vi "Tag Channel Example - Actually Right.vi"() -> ()   [LabVIEW 2023]
doc: "This VI demonstrates the fixes needed for the bugs that exist in the <b>Tag Channel Example - Almost Right.vi</b>."
uses:
  <extravilib>/ChannelInstances/Tag-u32/Instantiate.vi
  <extravilib>/ChannelInstances/Tag-u32/Endpoint.vi
  <extravilib>/ChannelInstances/Tag-u32/EndpointRead.vi
  <extravilib>/ChannelInstances/Tag-u32.lvlib
panel:
  out "C above threshold?":bool
  out "Thermometer C":dbl(slide) scale=0.0..10.0
  out "B above threshold?":bool
  out "Thermometer B":dbl(slide) scale=0.0..10.0
  out "A above threshold?":bool
  out "Thermometer A":dbl(slide) scale=0.0..10.0
  in  "Threshold Setting":u32(slide)=5 scale=0.0..10.0
  in  "Stop":bool
  # "Overview: Please review Tag Channel Example - Almost Right.vi before reviewing this VI.\n\nThis VI is identical to the other VI but with the two bugs fixed.\n\nInstructions:\n1. Run the VI. \n2. While running, change the Threshold Setting. Notice the thermometers immediately start using the new setting for their \"Too Hot\" indicators.\n3. Press the Stop button.\n4. Review the comments on the block diagram."
  # "When this VI is running, any time a thermometer is warmer than the Threshold Setting, that thermometer should say \"Too hot!\" in the Boolean at the bottom."
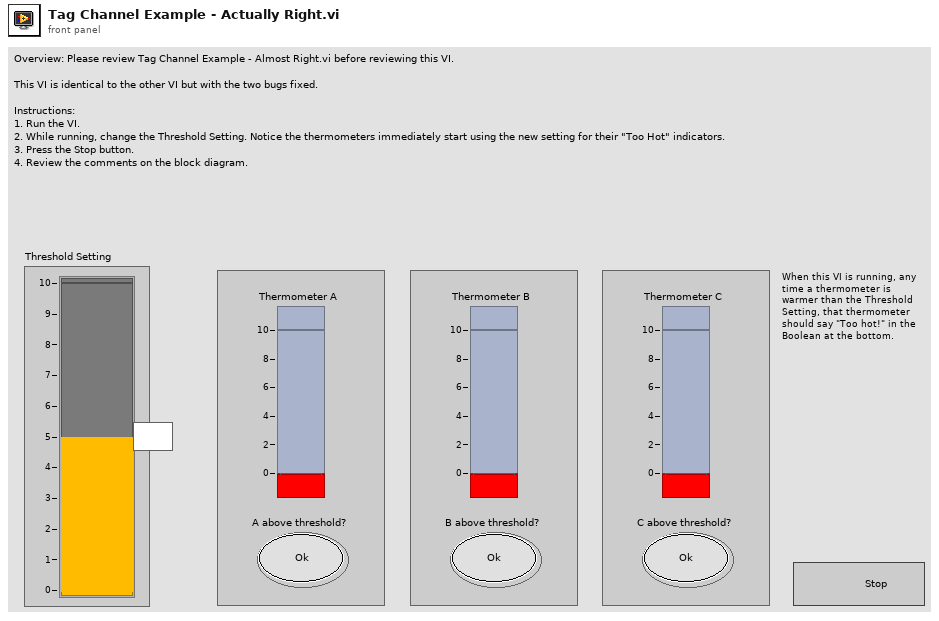
[diagram p1: front panel]
types:
  T1 = typedef "Tag-u32.lvlib/))Channel.ctl" = refnum<queue>
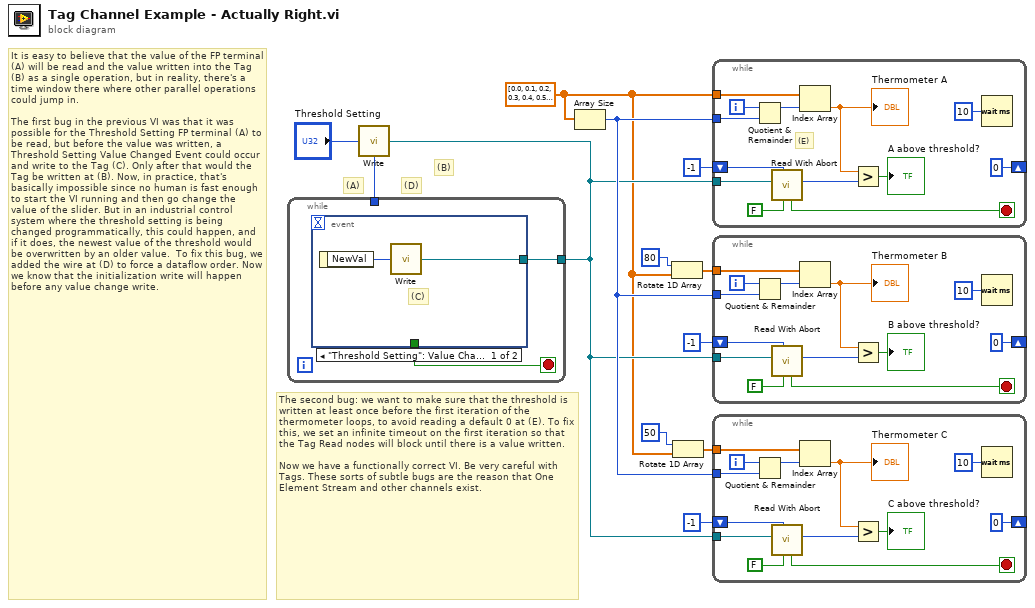
[diagram p0: block diagram]
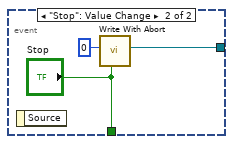
[diagram p2: hidden frame]
diagram:
  w7 = dbl[] [0.0, 0.1, 0.2, 0.3, 0.4, 0.5, 0.6, 0.7, 0.8, 0.9, 1.0, 1.1, 1.2, 1.3, 1.4, 1.5, 1.6, 1.7, 1.8, 1.9, 2.0, 2.1, 2.2, 2.3, 2.4, 2.5, 2.6, 2.7, 2.8, 2.9, 3.0, 3.1, 3.2, 3.3, 3.4, 3.5, 3.6, 3.7, 3.8, 3.9, 4.0, 4.1, 4.2, 4.3, 4.4, 4.5, 4.6, 4.7, 4.8, 4.9, 5.0, 5.1, 5.2, 5.3, 5.4, 5.5, 5.6, 5.7, 5.8, 5.9, 6.0, 6.1, 6.2, 6.3, 6.4, 6.5, 6.6, 6.7, 6.8, 6.9, 7.0, 7.1, 7.2, 7.3, 7.4, 7.5, 7.6, 7.7, 7.8, 7.9, 8.0, 8.1, 8.2, 8.3, 8.4, 8.5, 8.6, 8.7, 8.8, 8.9, 9.0, 9.1, 9.2, 9.3, 9.4, 9.5, 9.6, 9.7, 9.8, 9.9, 10.0, 10.0, 9.9, 9.8, 9.7, 9.6, 9.5, 9.4, 9.3, 9.2, 9.1, 9.0, 8.9, 8.8, 8.7, 8.6, 8.5, 8.4, 8.3, 8.2, 8.1, 8.0, 7.9, 7.8, 7.7, 7.6, 7.5, 7.4, 7.3, 7.2, 7.1, 7.0, 6.9, 6.8, 6.7, 6.6, 6.5, 6.4, 6.3, 6.2, 6.1, 6.0, 5.9, 5.8, 5.7, 5.6, 5.5, 5.4, 5.3, 5.2, 5.1, 5.0, 4.9, 4.8, 4.7, 4.6, 4.5, 4.4, 4.3, 4.2, 4.1, 4.0, 3.9, 3.8, 3.7, 3.6, 3.5, 3.4, 3.3, 3.2, 3.1, 3.0, 2.9, 2.8, 2.7, 2.6, 2.5, 2.4, 2.3, 2.2, 2.1, 2.0, 1.9, 1.8, 1.7, 1.6, 1.5, 1.4, 1.3, 1.2, 1.1, 1.0, 0.9, 0.8, 0.7, 0.6, 0.5, 0.4, 0.3, 0.2, 0.1, 0.0] ("x/y")
  # "The second bug: we want to make sure that the threshold is written at least once before the first iteration of the thermometer loops, to avoid reading a default 0 at (E). To fix this, we set an infinite timeout on the first iteration so that the Tag Read nodes will block until there is a value written.\n\nNow we have a functionally correct VI. Be very careful with Tags. These sorts of subtle bugs are the reason that One Element Stream and other channels exist."
  # "(D)"
  # "(B)"
  # "(A)"
  # "It is easy to believe that the value of the FP terminal (A) will be read and the value written into the Tag (B) as a single operation, but in reality, there's a time window there where other parallel operations could jump in.\n\nThe first bug in the previous VI was that it was possible for the Threshold Setting FP terminal (A) to be read, but before the value was written, a Threshold Setting Value Changed Event could occur and write to the Tag (C). Only after that would the Tag be written at (B). Now, in practice, that's basically impossible since no human is fast enough to start the VI running and then go change the value of the slider. But in an industrial control system where the threshold setting is being changed programmatically, this could happen, and if it does, the newest value of the threshold would be overwritten by an older value.  To fix this bug, we added the wire at (D) to force a dataflow order. Now we know that the initialization write will happen before any value change write."
  n1 = call <extravilib>:"Write.vi"("element"="Threshold Setting") -> ("previous element"=w4:u32, "channel"=w10:T1)
  n2 = while {
    tunnel: w10 -> [w14]
    tunnel: w4 -> [_]
    stop <- w13 stop-if-true
    n3 = event shown="[0] \"Threshold Setting\": Value Change" {
      selector: _ -> [_ _]
      dyn-events: _ -> [_ _]
      timeout: _ -> [_ _]
      tunnel: [w16 w19] -> w14
      tunnel: [_ "Stop"] -> w13
      event "Threshold Setting": Value Change {
        # "(C)"
        n4 = event-data() -> ("NewVal"=w15:u32)  [unwired: 1 in]
        n5 = call <extravilib>:"Write.vi"("element"=w15) -> ("channel"=w16:T1)  [unwired: 1 out]
      }
      event "Stop": Value Change {
        n6 = event-data() -> ()  [unwired: 1 in, 1 out]
        n7 = call <extravilib>:"Write With Abort.vi"("abort"="Stop", "element"=u32 0) -> ("channel"=w19:T1)  [unwired: 7 in, 2 out]
      }
    }
  }
  n8 = Array Size(array=w7) -> (size(s)=w11:i32)
  n9 = Rotate 1D Array(1:w7, 2:80 ("n")) -> (0:w6:dbl[])
  n10 = Rotate 1D Array(1:w7, 2:50 ("n")) -> (0:w9:dbl[])
  n11 = while {
    tunnel: w10 -> [w32]
    tunnel: w11 -> [w26]
    tunnel: w7 -> [w25]
    shift-right: [0 ("timeout in ms (0)")] -> _
    shift-left: -1 ("timeout in ms (0)") -> [w21]
    i -> [w27]
    stop <- w31 stop-if-true
    # "(E)"
    n12 = Quotient & Remainder(x=w27, y=w26) -> (x-y*floor(x/y)=w24:i32)  [unwired: 1 out]
    n13 = call <extravilib>:"Read With Abort.vi"("abort"=FALSE, "timeout in ms (0)"=w21, "channel"=w32) -> ("element"=w30:u32, "aborted?"=w31:bool)  [unwired: 6 in, 1 out]
    n14 = Index Array(array=w25, index=w24) -> (element=w23:dbl)
    "Thermometer A" <- w23
    n15 = Greater?(x=w23, y=w30) -> (0:→"A above threshold?":bool)
    n16 = Wait (ms)(milliseconds to wait=u32 10) -> ()  [unwired: 1 out]
  }
  n17 = while {
    tunnel: w10 -> [w45]
    tunnel: w11 -> [w40]
    tunnel: w6 -> [w39]
    shift-right: [0 ("timeout in ms (0)")] -> _
    shift-left: -1 ("timeout in ms (0)") -> [w33]
    i -> [w41]
    stop <- w44 stop-if-true
    n18 = Quotient & Remainder(x=w41, y=w40) -> (x-y*floor(x/y)=w38:i32)  [unwired: 1 out]
    n19 = call <extravilib>:"Read With Abort.vi"("abort"=FALSE, "timeout in ms (0)"=w33, "channel"=w45) -> ("element"=w43:u32, "aborted?"=w44:bool)  [unwired: 6 in, 1 out]
    n20 = Index Array(array=w39, index=w38) -> (element=w36:dbl)
    "Thermometer B" <- w36
    n21 = Greater?(x=w36, y=w43) -> (0:→"B above threshold?":bool)
    n22 = Wait (ms)(milliseconds to wait=u32 10) -> ()  [unwired: 1 out]
  }
  n23 = while {
    tunnel: w10 -> [w58]
    tunnel: w11 -> [w53]
    tunnel: w9 -> [w52]
    shift-right: [0 ("timeout in ms (0)")] -> _
    shift-left: -1 ("timeout in ms (0)") -> [w47]
    i -> [w54]
    stop <- w57 stop-if-true
    n24 = Quotient & Remainder(x=w54, y=w53) -> (x-y*floor(x/y)=w51:i32)  [unwired: 1 out]
    n25 = call <extravilib>:"Read With Abort.vi"("abort"=FALSE, "timeout in ms (0)"=w47, "channel"=w58) -> ("element"=w56:u32, "aborted?"=w57:bool)  [unwired: 6 in, 1 out]
    n26 = Index Array(array=w52, index=w51) -> (element=w49:dbl)
    "Thermometer C" <- w49
    n27 = Greater?(x=w49, y=w56) -> (0:→"C above threshold?":bool)
    n28 = Wait (ms)(milliseconds to wait=u32 10) -> ()  [unwired: 1 out]
  }
